vi "Stage Scanning Cambridge V1.vi"() -> ()   [LabVIEW 2016]
uses:
  <vilib>/rvi/DataTransferAndStorage/Container/XNode/niFpgaContainer.xnode
  <vilib>/Platform/TimedLoop/XDataNode/wakeup.ctl
  <vilib>/Platform/TimedLoop/XDataNode/XDNodeRunTimeDep.lvlib
  <vilib>/Platform/TimedLoop/XDataNode/nitl_modes.ctl
  <vilib>/Platform/TimedLoop/XDataNode/timing_clust.ctl
  <vilib>/Platform/TimedLoop/XDataNode/XDataNode.xnode
  <vilib>/eio/EIONode/EIONode.xnode
  <vilib>/rvi/eio/common/nirviEmuTemplateMethod_errors.vi
  <vilib>/rvi/Memory/Memory_Emulation/nirvimemoryFastEmulation.vi
  <vilib>/rvi/Memory/Memory_Emulation/nirvimemoryEmulation.vi
  <vilib>/rvi/FIFO/Fifo_Resource/nirvififoEmulationRead.vi
  <vilib>/rvi/FIFO/Fifo_Resource/nirvififoEmulationWrite.vi
  <vilib>/rvi/interface/RandomDataEmulation/nirviRandomDataFpgaReadWriteTemplate.vi
panel:
  in  "APD Number":i32
  in  "Trigger Delay":u32
  in  "Dead Lines":u16
  in  "Pixels Per Line":i32
  out "Ready For Write":bool
  in  "Cycles Per Pixel":u32
  # "Copyright (C) 2020 Edward S Allgeyer\n\nRedistribution and use in source and binary forms, with or without\nmodification, are permitted provided that the following conditions\nare met:\n\n1. Redistributions of source code must retain the above copyright\n   notice, this list of conditions and the following disclaimer.\n\n2. Redistributions in binary form must reproduce the above copyright\n   notice, this list of conditions and the following disclaimer in\n   the documentation and/or other materials provided with the\n   distribution.\n\n3. Neither the name of the copyright holder nor the names of its\n   contributors may be used to endorse or promote products derived\n   from this software without specific prior written permission.\n\nTHIS SOFTWARE IS PROVIDED BY THE COPYRIGHT HOLDERS AND CONTRIBUTORS\n\"AS IS\" AND ANY EXPRESS OR IMPLIED WARRANTIES, INCLUDING, BUT NOT\nLIMITED TO, THE IMPLIED WARRANTIES OF MERCHANTABILITY AND FITNESS\nFOR A PARTICULAR PURPOSE ARE DISCLAIMED. IN NO EVENT SHALL THE\nCOPYRIGHT HOLDER OR CONTRIBUTORS BE LIABLE FOR ANY DIRECT, INDIRECT,\nINCIDENTAL, SPECIAL, EXEMPLARY, OR CONSEQUENTIAL DAMAGES (INCLUDING,\nBUT NOT LIMITED TO, PROCUREMENT OF SUBSTITUTE GOODS OR SERVICES;\nLOSS OF USE, DATA, OR PROFITS; OR BUSINESS INTERRUPTION) HOWEVER\nCAUSED AND ON ANY THEORY OF LIABILITY, WHETHER IN CONTRACT, STRICT\nLIABILITY, OR TORT (INCLUDING NEGLIGENCE OR OTHERWISE) ARISING IN\nANY WAY OUT OF THE USE OF THIS SOFTWARE, EVEN IF ADVISED OF THE\nPOSSIBILITY OF SUCH DAMAGE."
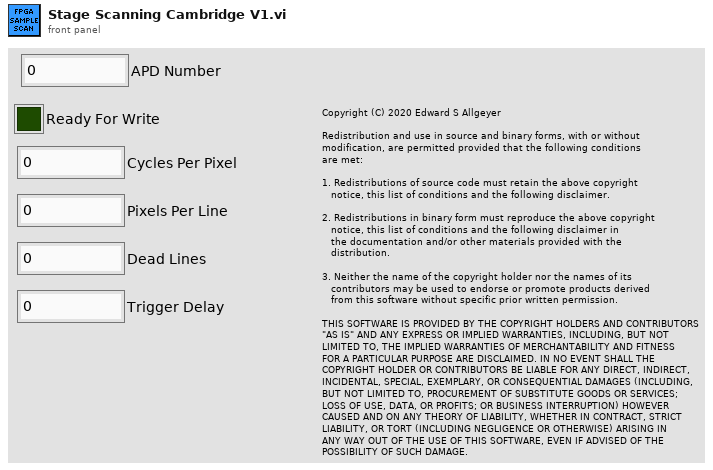
[diagram p1: front panel]
types:
  T1 = typedef "XDNodeRunTimeDep.lvlib/timing_clust.ctl" = cluster{"Expected End [f-1]":u64, "Actual End [f-1]":u64, "Finished Late? [f-1]":bool, "Expected End [i-1]":u64, "Actual End [i-1]":u64, "Finished Late? [i-1]":bool, "Expected Start [i]":u64, "Actual Start [i]":u64, "Expected Start [f]":u64, "Actual Start [f]":u64, "Source Name":string, "Structure Name":string, "Period":i64, "Deadline":i64, "Offset":i64, "Start":i64, "Priority":i32, "Timeout":i32, "Mode":T2, "Wakeup Reason":T3, "Error":errorcluster, "Source Type":string, "Secondary Source Type":string, "Global End Time":u64, "Global Start Time":u64, "Frame Duration":u64, "Iteration Duration":u64, "Assigned CPU":i32, "I/O Scan Engine Mode":u32}
  T2 = typedef "XDNodeRunTimeDep.lvlib/nitl_modes.ctl" = enum32{"No Change", "Process missed periods, maintain original phase", "Discard missed periods, maintain original phase", "Process missed periods, ignore original phase", "Discard missed periods, ignore original phase"}
  T3 = typedef "XDNodeRunTimeDep.lvlib/wakeup.ctl" = enum32{"Normal", "Aborted", "Asynchronous wakeup", "Timing source error", "Timed loop error", "Timeout"}
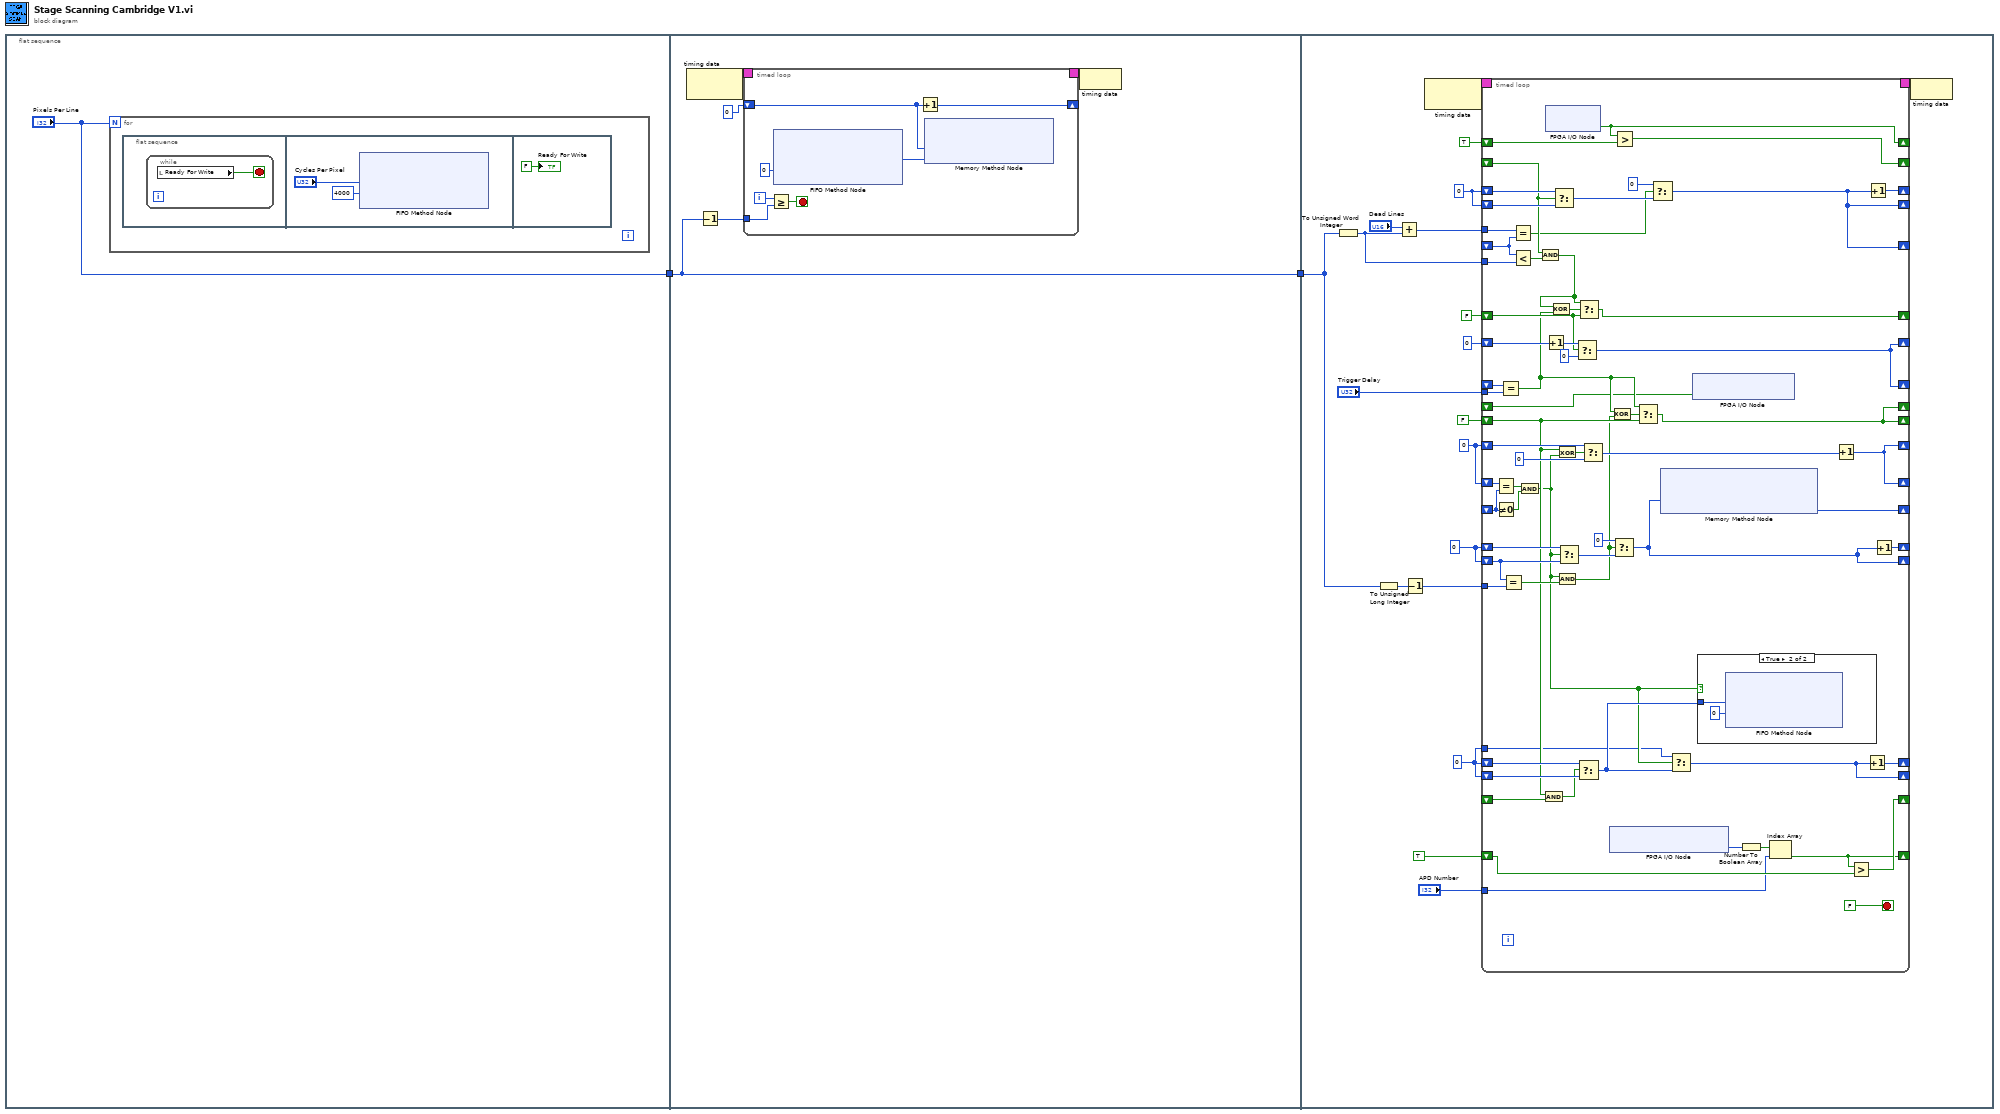
[diagram p0: block diagram]
diagram:
  n1 = flat-sequence {
    tunnel: ["Pixels Per Line"] -> w2
    tunnel: w2 -> [w9]
    tunnel: [w9] -> w1
    tunnel: w1 -> [w25]
    frame #0 {
      n2 = for {
        N: "Pixels Per Line" -> [_]
        n3 = flat-sequence {
          frame #0 {
            n4 = while {
              stop <- w4 stop-if-true
              n5 = local read "Ready For Write"() -> (w4:bool)
            }
          }
          frame #1 {
            n6 = xnode ("FIFO Method Node")("Element"="Cycles Per Pixel", "Timeout"=4000) -> ()  [unwired: 1 in, 2 out]
          }
          frame #2 {
            "Ready For Write" <- FALSE ("Ready For Write (SLOW)")
          }
        }
      }
    }
    frame #1 {
      n7 = node-c288() -> (w12:T1)  [unwired: 1 in]
      n8 = Decrement(x=w9) -> (x-1=w8:i32)
      n9 = timed-loop {
        timing: w12 -> [_]
        timing-out: [_] -> w11
        shift-right: [w17] -> _
        shift-left: u32 0 -> [w15]
        tunnel: w8 -> [w13]
        i -> [w16]
        stop <- w19 stop-if-true
        n10 = Greater Or Equal?(x=w16, y=w13) -> (x >= y?=w19:bool)
        n11 = xnode ("FIFO Method Node")("Timeout"=0) -> ("Element"=w14:u32)  [unwired: 1 in, 2 out]
        n12 = Increment(x=w15) -> (x+1=w17:u32)
        n13 = xnode ("Memory Method Node")("Address"=w15, "Data"=w14) -> ()  [unwired: 1 in, 1 out]
      }
      n14 = node-c288(w11) -> ()
    }
    frame #2 {
      w35 = u16 0
      w24 = u64 0
      w28 = u32 0
      w29 = u32 0
      n15 = To Unsigned Word Integer(number=w25) -> (unsigned 16bit integer=w40:u16)
      n16 = To Unsigned Long Integer(number=w25) -> (unsigned 32bit integer=w33:u32)
      n17 = Add(x="Dead Lines", y=w40) -> (x+y=w37:u16)
      n18 = Decrement(x=w33) -> (x-1=w27:u32)
      n19 = node-c288() -> (w42:T1)  [unwired: 1 in]
      n20 = timed-loop {
        shift-right: [w98] -> _
        shift-left: w29 -> [w107]
        shift-right: [w98] -> _
        shift-left: w29 -> [w104]
        shift-right: [w103] -> _
        shift-left: w28 -> [w97]
        shift-right: [w74] -> _
        shift-left: w28 -> [w95]
        shift-right: [w73] -> _
        shift-left: _ -> [w55]
        tunnel: w27 -> [w96]
        shift-right: [w45] -> _
        shift-left: FALSE -> [w72]
        shift-right: [w93] -> _
        shift-left: w24 -> [w88]
        shift-right: [w75] -> _
        shift-left: _ -> [w90]
        shift-right: [w89] -> _
        shift-left: w24 -> [w92]
        shift-right: [w86] -> _
        shift-left: FALSE -> [w81]
        shift-right: [w83] -> _
        shift-left: u32 0 -> [w85]
        shift-right: [w83] -> _
        shift-left: _ -> [w80]
        tunnel: "Trigger Delay" -> [w79]
        shift-right: [w46] -> _
        shift-left: _ -> [w60]
        shift-right: [w77] -> _
        shift-left: TRUE -> [w78]
        timing: w42 -> [_]
        timing-out: [_] -> w41
        shift-right: [w48] -> _
        shift-left: TRUE -> [w76]
        shift-right: [w65] -> _
        shift-left: w35 -> [w69]
        shift-right: [w64] -> _
        shift-left: w35 -> [w68]
        shift-right: [w64] -> _
        shift-left: _ -> [w62]
        tunnel: w37 -> [w63]
        tunnel: w40 -> [w61]
        tunnel: "APD Number" -> [w49]
        shift-right: [w45] -> _
        shift-left: _ -> [w44]
        tunnel: w24 -> [w43]
        stop <- FALSE stop-if-true
        n21 = Equal?(x=w104, y=w55) -> (x = y?=w54:bool)
        n22 = Not Equal To 0?(x=w55) -> (x != 0?=w53:bool)
        n23 = Equal?(x=w80, y=w79) -> (x = y?=w70:bool)
        n24 = Equal?(x=w95, y=w96) -> (x = y?=w94:bool)
        n25 = Equal?(x=w63, y=w62) -> (x = y?=w57:bool)
        n26 = Less?(x=w62, y=w61) -> (x < y?=w59:bool)
        n27 = And(x=w54, y=w53) -> (x .and. y?=w52:bool)
        n28 = And(x=w60, y=w59) -> (x .and. y?=w58:bool)
        n29 = And(x=w72, y=w90) -> (x .and. y?=w91:bool)
        n30 = xnode "FPGA I/O Node"() -> ("RTSI0"=w77:bool)  [unwired: 1 in, 1 out]
        n31 = Increment(x=w85) -> (x+1=w84:u32)
        n32 = Exclusive Or(1:w70, 2:w58) -> (0:w87:bool)
        n33 = Select(t=w69, s=w60, f=w68) -> (s? t:f=w67:u16)
        n34 = Exclusive Or(1:w52, 2:w72) -> (0:w105:bool)
        n35 = And(x=w52, y=w94) -> (x .and. y?=w56:bool)
        n36 = Select(t=w97, s=w52, f=w95) -> (s? t:f=w102:u32)
        n37 = Select(t=w84, s=w81, f=u32 0) -> (s? t:f=w83:u32)
        n38 = Select(t=w88, s=w91, f=w92) -> (s? t:f=w71:u64)
        n39 = Select(t=w58, s=w87, f=w81) -> (s? t:f=w86:bool)
        n40 = Select(t=w107, s=w105, f=u32 0) -> (s? t:f=w99:u32)
        n41 = xnode "FPGA I/O Node"() -> ("Connector1/DIOPORT0"=w51:u8)  [unwired: 1 in, 1 out]
        n42 = Exclusive Or(1:w56, 2:w70) -> (0:w100:bool)
        n43 = Select(t=u32 0, s=w56, f=w102) -> (s? t:f=w74:u32)
        n44 = Greater?(x=w77, y=w78) -> (0:w46:bool)
        n45 = Select(t=w70, s=w100, f=w72) -> (s? t:f=w45:bool)
        n46 = Select(t=u16 0, s=w57, f=w67) -> (s? t:f=w64:u16)
        n47 = xnode ("Memory Method Node")("Address"=w74) -> ("Data"=w73:u32)  [unwired: 1 in, 1 out]
        n48 = Select(t=w43, s=w52, f=w71) -> (s? t:f=w89:u64)
        n49 = xnode "FPGA I/O Node"("Connector1/DIO15"=w44) -> ()  [unwired: 1 in, 1 out]
        n50 = case shown="True" w52 {
          tunnel: w71 -> [_ w108]
          frame False {
          }
          frame True {
            n51 = xnode ("FIFO Method Node")("Element"=w108, "Timeout"=0) -> ()  [unwired: 1 in, 2 out]
          }
        }
        n52 = Number To Boolean Array(number=w51) -> (Boolean array=w50:bool[])
        n53 = Index Array(array=w50, index=w49) -> (element=w48:bool)
        n54 = Increment(x=w99) -> (x+1=w98:u32)
        n55 = Greater?(x=w48, y=w76) -> (0:w75:bool)
        n56 = Increment(x=w89) -> (x+1=w93:u64)
        n57 = Increment(x=w64) -> (x+1=w65:u16)
        n58 = Increment(x=w74) -> (x+1=w103:u32)
      }
      n59 = node-c288(w41) -> ()
    }
  }
